vi "Open.vi"(8 "error in (no error)":errorcluster, 11 "Text File Sink in":refnum<class "Text File Sink.lvclass">) -> (0 "error out":errorcluster, 3 "Text File Sink out":refnum<class "Text File Sink.lvclass">)   [LabVIEW 2020, in "MVA Framework.lvlib" / "Text File Sink.lvclass"]
doc: "--\nCopyright © 2017 Composed SystemsI All rights reserved.\n\nAuthor: Jon McBee <jon.mcbee@composed.io>\n\nThis library is provided \"AS IS\" ,WITHOUT WARRANTIES OR\nCONDITIONS OF ANY KIND, either express or implied.\n\nComposed Systems -- composed.io\n\nStream 0.0.1.1\nJon McBee - Composed Systems\nCopyright (c) 2017, Composed Systems"
uses:
  Text File Sink.lvclass
  Text File Sink.lvclass/Text File Sink.ctl
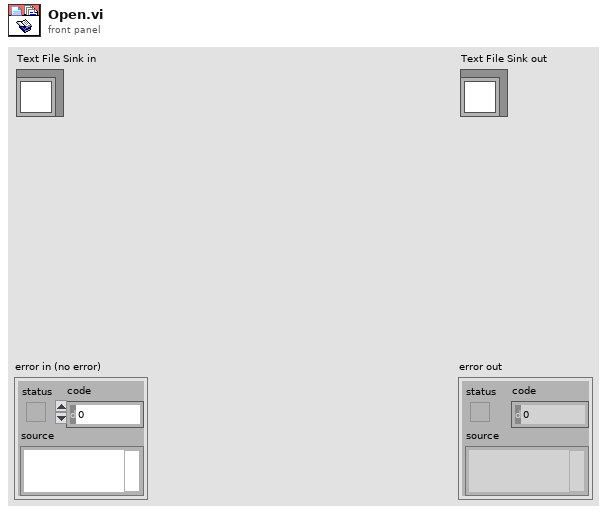
[diagram p1: front panel]
types:
  T1 = enum16{"open", "replace", "create", "open or create", "replace or create", "replace or create with confirmation"}
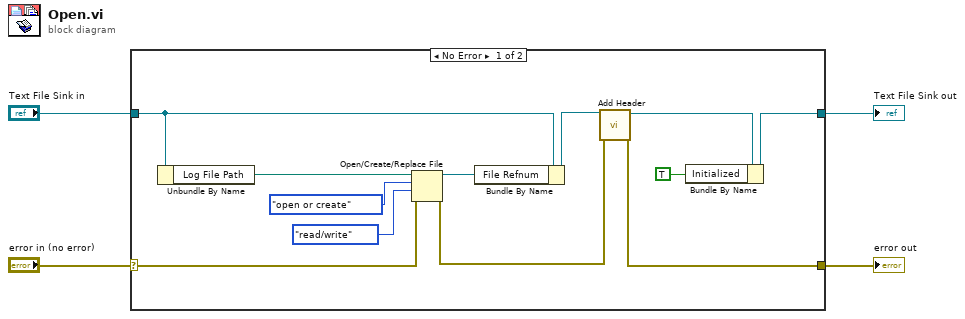
[diagram p0: block diagram]
diagram:
  n1 = case shown="No Error" "error in (no error)" {
    selector: "error in (no error)" -> [w15 w18]
    tunnel: [w11 w18] -> w3
    tunnel: [w9 w17] -> w1
    tunnel: "Text File Sink in" -> [w7 w17]
    frame No Error {
      n2 = Unbundle By Name(w7) -> ("Log File Path"=w16:path)
      n3 = Open/Create/Replace File(file path (use dialog)=w16, error in=w15, operation (0:open)=T1."open or create", access (0:read/write)=enum16{"read/write", "read-only", "write-only"}."read/write") -> (refnum out=w12:refnum<file>, error out=w5:errorcluster)  [unwired: 2 in, 1 out]
      n4 = Bundle By Name(cluster=w7, "File Refnum"=w12) -> (w6:refnum<class "Text File Sink.lvclass">)
      n5 = call-dynamic "Add Header.vi"("error in (no error)"=w5, "Text File Sink in"=w6) -> ("error out"=w11:errorcluster, "Text File Sink out"=w10:refnum<class "Text File Sink.lvclass">)  [unwired: 8 in]
      n6 = Bundle By Name(cluster=w10, "Initialized"=TRUE) -> (w9:refnum<class "Text File Sink.lvclass">)
    }
    frame Error {
    }
  }
  "error out" <- w3
  "Text File Sink out" <- w1
